vi "createILCADC.vi"(8 "error in (no error)":errorcluster, 10 "Channel":u8, 11 "IILCADCFactory in":refnum<class "IILCADCFactory.lvclass">) -> (0 "error out":errorcluster, 2 "ILCADC":refnum<class "IILCADC.lvclass">, 3 "IILCADCFactory out":refnum<class "IILCADCFactory.lvclass">)   [LabVIEW 2015, in "IILCADCFactory.lvclass"]
uses:
  IILCADCFactory.lvclass
  ILCADC/IILCADC/IILCADC.lvclass
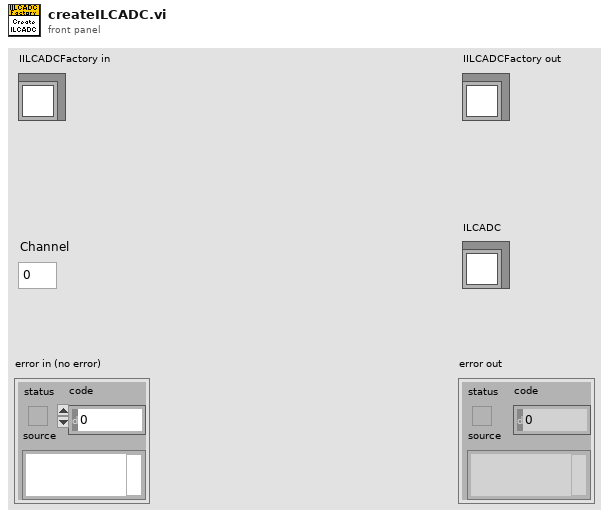
[diagram p1: front panel]
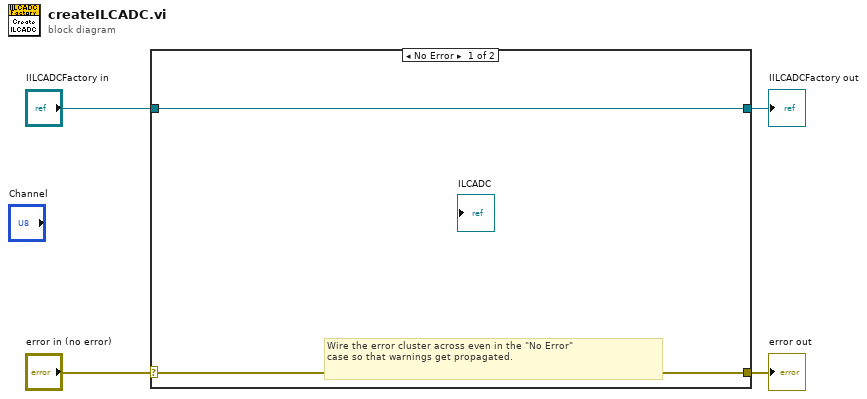
[diagram p0: block diagram]
diagram:
  n1 = case shown="No Error" "error in (no error)" {
    selector: "error in (no error)" -> [w5 w8]
    tunnel: [w5 w8] -> w3
    tunnel: [w6 w7] -> w1
    tunnel: "IILCADCFactory in" -> [w6 w7]
    frame No Error {
      # "Wire the error cluster across even in the \"No Error\"\ncase so that warnings get propagated."
    }
    frame Error {
    }
  }
  "error out" <- w3
  "IILCADCFactory out" <- w1
